vi "dfd_Group Delay_Gradient Design.vi"(4 "radius":dbl=1.0, 5 "parameters":T1={"iteration"={"epsilon"=1e-05, "times"=300}, "initial guess"={"iteration times"=5, "seed"=1.0}}, 6 "fs (Hz)":dbl=1.0, 7 "integer tau?":bool=TRUE, 8 "error in (no error)":errorcluster, 9 "P":i32=2, 10 "band specification":T3[](array[typedef]) {"subband specs"."weight" format="%.2f"}, 11 "order":i32) -> (0 "error out":errorcluster, 1 "Error":dbl, 2 "Coefficients":cluster{"r":dbl[], "theta":dbl[], "offset":dbl}, 3 "Design Info":T2={"p"=2, "freq grid"=[], "d"=[], "weight"=[], "Order"=0, "radius"=1.0})   [LabVIEW 2017, in "NI_DigFilter_Design.lvlib"]
uses:
  <vilib>/addons/Digital Filter Design/NI_DigFilter_Design.lvlib
  <vilib>/addons/Digital Filter Design/_GroupDelay.llb/dfd_Group Delay_Band Spec.ctl
  <vilib>/addons/Digital Filter Design/_GroupDelay.llb/dfd_Group Delay_Design Info.ctl
  <vilib>/addons/Digital Filter Design/NI_DigFilterLicensed.lvlib
panel:
  # "freq"
  # "group delay"
  # "weight"
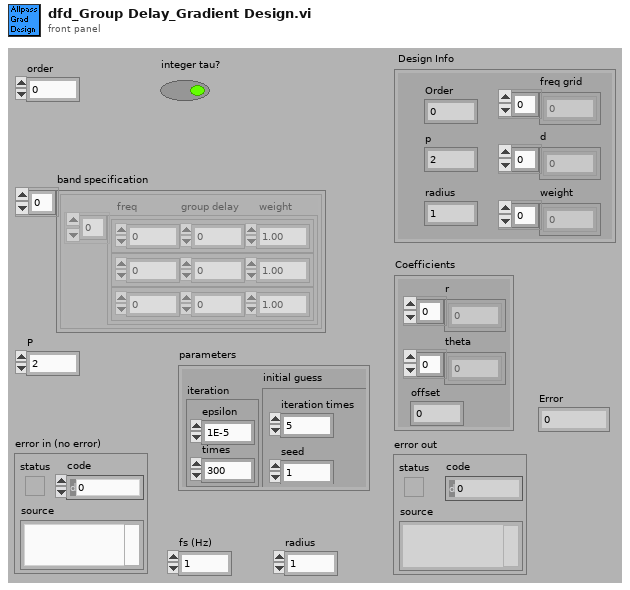
[diagram p1: front panel]
types:
  T1 = cluster{"iteration":cluster{"epsilon":dbl, "times":i32}, "initial guess":cluster{"iteration times":i32, "seed":dbl}}
  T2 = typedef "dfd_Group Delay_Design Info.ctl" = cluster{"p":i32, "freq grid":dbl[], "d":dbl[], "weight":dbl[], "Order":i32, "radius":dbl}
  T3 = typedef "NI_DigFilterLicensed.lvlib/dfd_Group Delay_Band Spec.ctl" = cluster{"subband specs":cluster{"freq":dbl, "group delay":dbl, "weight":dbl}[]}
  T4 = cluster{"r":dbl[], "theta":dbl[], "offset":dbl}[]
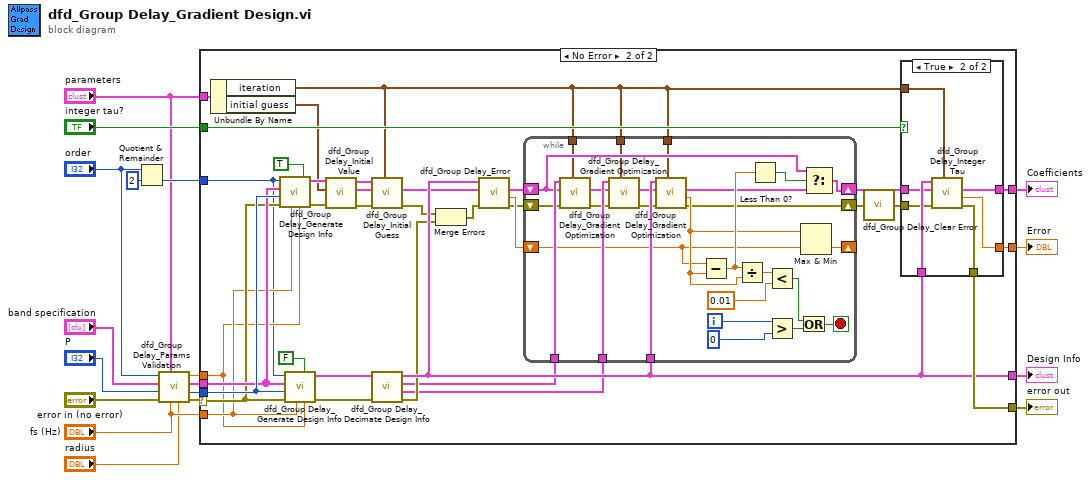
[diagram p0: block diagram]
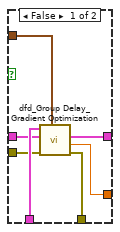
[diagram p3: hidden frame]
diagram:
  n1 = Quotient & Remainder(x="order", y=2) -> (floor(x/y)=w2:i32)  [unwired: 1 out]
  n2 = call <vilib>:"dfd_Group Delay_Params Validation.vi"("max pole radius (in)"="radius", "fs [Hz]"="fs (Hz)", "parameters"="parameters", "error in (no error)"="error in (no error)", "p (in)"="P", "dfd_Group Delay_Band Spec"="band specification", "order"="order") -> ("error out"=w13:errorcluster, "p (out)"=w11:i32, "dfd_Group Delay_Band Spec (dup)"=w9:T3[], "max pole radius (out)"=w5:dbl)  [unwired: 1 out]
  n3 = case shown="No Error" w13 {
    selector: w13 -> [w19 w41]
    tunnel: [_ w51] -> w18
    tunnel: [_ w50] -> w4
    tunnel: "integer tau?" -> [_ w49]
    tunnel: [_ w33] -> w16
    tunnel: [w19 w46] -> w15
    tunnel: w11 -> [_ w43]
    tunnel: w9 -> [_ w42]
    tunnel: "fs (Hz)" -> [_ w40]
    tunnel: w5 -> [_ w39]
    tunnel: w2 -> [_ w28]
    tunnel: "parameters" -> [_ w22]
    frame Error {
    }
    frame No Error {
      n4 = Unbundle By Name(w22) -> ("iteration"=w20:cluster{"epsilon":dbl, "times":i32}, "initial guess"=w21:cluster{"iteration times":i32, "seed":dbl})
      n5 = call <vilib>:"dfd_Group Delay_Generate Design Info.vi"("radius"=w39, "Add Band?"=TRUE, "fs [Hz]"=w40, "error in (no error)"=w41, "p"=w43, "band specification"=w42, "order"=w28) -> ("error out"=w44:errorcluster, "Group Delay Design Info"=w45:T2)  [unwired: 1 in, 2 out]
      n6 = call <vilib>:"dfd_Group Delay_Generate Design Info.vi"("radius"=w39, "Add Band?"=FALSE, "fs [Hz]"=w40, "error in (no error)"=w41, "p"=w43, "band specification"=w42, "order"=w28) -> ("error out"=w32:errorcluster, "Group Delay Design Info"=w34:T2)  [unwired: 1 in, 2 out]
      n7 = call <vilib>:"dfd_Group Delay_Initial Value.vi"("error in (no error)"=w44, "initial guess"=w21, "Design Info"=w45) -> ("error out"=w25:errorcluster, "Coefficients"=w26:T4, "Design Info (dup)"=w27:T2)  [unwired: 6 out]
      n8 = call <vilib>:"dfd_Group Delay_Initial Guess.vi"("parameter"=w20, "error in (no error)"=w25, "Coefficients (array)"=w26, "Design Info"=w27) -> ("error out"=w24:errorcluster, "Coefficients (out)"=w23:cluster{"r":dbl[], "theta":dbl[], "offset":dbl})  [unwired: 6 out]
      n9 = call <vilib>:"dfd_Group Delay_Decimate Design Info.vi"("error in (no error)"=w32, "Group Delay Design Info (in)"=w34) -> ("error out"=w31:errorcluster, "Group Delay Design Info (even)"=w29:T2, "Group Delay Design Info (odd)"=w30:T2, "Group Delay Design Info (dup)"=w33:T2)  [unwired: 6 out]
      n10 = Merge Errors(w24, w31) -> (w38:errorcluster)
      n11 = call <vilib>:"dfd_Group Delay_Error.vi"("error in (no error)"=w38, "Coefficients"=w23, "Design Info"=w33) -> ("error out"=w47:errorcluster, "Error"=w52:dbl, "Coefficients (dup)"=w37:cluster{"r":dbl[], "theta":dbl[], "offset":dbl})  [unwired: 6 out]
      n12 = while {
        shift-right: [w76] -> _
        shift-left: w52 -> [w77]
        shift-right: [w79] -> w48
        shift-left: w37 -> [w81]
        tunnel: w30 -> [w88]
        tunnel: w33 -> [w87]
        tunnel: w29 -> [w86]
        shift-right: [w75] -> w36
        shift-left: w47 -> [w72]
        tunnel: w20 -> [w74]
        tunnel: w20 -> [w73]
        tunnel: w20 -> [w70]
        i -> [w93]
        stop <- w89 stop-if-true
        n13 = call <vilib>:"dfd_Group Delay_Gradient Optimization.vi"("parameter"=w70, "error in (no error)"=w72, "Coefficients (in)"=w81, "Design Info"=w88) -> ("error out"=w71:errorcluster, "Coefficients (out)"=w85:cluster{"r":dbl[], "theta":dbl[], "offset":dbl})  [unwired: 2 in, 4 out]
        n14 = call <vilib>:"dfd_Group Delay_Gradient Optimization.vi"("parameter"=w74, "error in (no error)"=w71, "Coefficients (in)"=w85, "Design Info"=w86) -> ("error out"=w69:errorcluster, "Coefficients (out)"=w84:cluster{"r":dbl[], "theta":dbl[], "offset":dbl})  [unwired: 2 in, 4 out]
        n15 = call <vilib>:"dfd_Group Delay_Gradient Optimization.vi"("parameter"=w73, "error in (no error)"=w69, "Coefficients (in)"=w84, "Design Info"=w87) -> ("error out"=w75:errorcluster, "Error"=w78:dbl, "Coefficients (out)"=w80:cluster{"r":dbl[], "theta":dbl[], "offset":dbl})  [unwired: 2 in, 3 out]
        n16 = Subtract(x=w77, y=w78) -> (x-y=w83:dbl)
        n17 = Divide(x=w83, y=w78) -> (x/y=w95:dbl)
        n18 = Less Than 0?(x=w83) -> (x < 0?=w82:bool)
        n19 = Less?(x=w95, y=0.01) -> (x < y?=w91:bool)
        n20 = Greater?(x=w93, y=0) -> (0:w90:bool)
        n21 = Or(x=w91, y=w90) -> (x .or. y?=w89:bool)
        n22 = Max & Min(x=w78, y=w77) -> (min(x,y)=w76:dbl)  [unwired: 1 out]
        n23 = Select(t=w81, s=w82, f=w80) -> (s? t:f=w79:cluster{"r":dbl[], "theta":dbl[], "offset":dbl})
      }
      n24 = call <vilib>:"dfd_Group Delay_Clear Error.vi"("error in (no error)"=w36) -> ("error out"=w35:errorcluster)
      n25 = case shown="True" w49 {
        tunnel: [w56 w65] -> w51
        tunnel: w48 -> [w60 w67]
        tunnel: [w59 w66] -> w50
        tunnel: w33 -> [w61 w68]
        tunnel: w35 -> [w58 w62]
        tunnel: [w57 w64] -> w46
        tunnel: w20 -> [w55 w63]
        frame False {
          n26 = call <vilib>:"dfd_Group Delay_Gradient Optimization.vi"("parameter"=w55, "error in (no error)"=w58, "Coefficients (in)"=w60, "Design Info"=w61) -> ("error out"=w57:errorcluster, "Error"=w56:dbl, "Coefficients (out)"=w59:cluster{"r":dbl[], "theta":dbl[], "offset":dbl})  [unwired: 2 in, 3 out]
        }
        frame True {
          n27 = call <vilib>:"dfd_Group Delay_Integer Tau.vi"("parameter"=w63, "error in (no error)"=w62, "Coefficients (in)"=w67, "Design Info"=w68) -> ("error out"=w64:errorcluster, "Error"=w65:dbl, "Coefficients (out)"=w66:cluster{"r":dbl[], "theta":dbl[], "offset":dbl})  [unwired: 5 out]
        }
      }
    }
  }
  "Design Info" <- w16
  "Error" <- w18
  "error out" <- w15
  "Coefficients" <- w4
